vi "Swerve Drive.vi"(0 "X":dbl, 1 "Rot. Point X":dbl, 3 "Rot. Point Y":dbl, 5 "Y":dbl, 7 "Z":dbl, 11 "Error In":errorcluster, 12 "Robot Centric?":bool=TRUE, 13 "Autonomous?":bool, 14 "Yaw":dbl) -> (4 "Front Left Output":dbl, 6 "Front Right Output":dbl, 8 "Back Left Output":dbl, 10 "Back Right Output":dbl, 15 "Error Out":errorcluster)   [LabVIEW 2018]
uses:
  <vilib>/Rock Robotics/WPI/ThirdParty/Phoenix-LabVIEW/Motor Controller/Controls/CTRE_Phoenix_MotorControl_ControlMode.ctl
panel:
  in  "Robot Length":dbl=33.5
  in  "Robot Width":dbl=28.5
  # "Swerve Drive Teleoperated Control\nFRC Team 34"
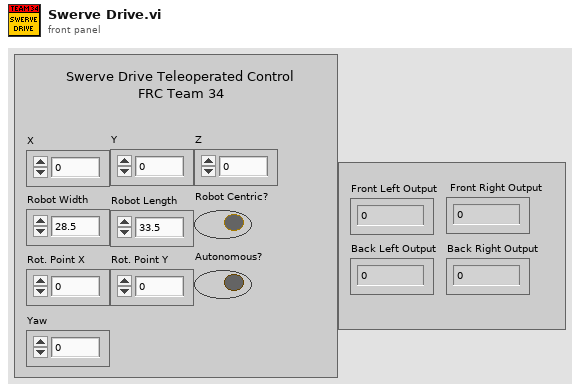
[diagram p1: front panel]
types:
  T1 = enum16{"Front Left", "Front Right", "Back Left", "Back Right"}
  T2 = typedef "CTRE_Phoenix_MotorControl_ControlMode.ctl" = u16
  T3 = typedef "WPI_MotorControlDeviceRef.ctl" = cluster{"DeviceStatus":errorcluster, "Type":T4, "PWM":cluster{"PWM Channel":T5, "DeadBand":T6}, "CAN":cluster{"Device Number":u8, "SetOutput VI Ref":variant, "GetOutput VI Ref":variant, "Enable VI Ref":variant, "Disable VI Ref":variant, "Data":variant}, "Invert":bool, "DIO PWM":cluster{"PWM \"Enable\" Channel":T5, "DIOChannel":T7, "PWM Rate":dbl}}
  T4 = typedef "WPI_MotorControlType.ctl" = enum16{"PWM", "CAN", "DIO PWM"}
  T5 = typedef "FPGA_DIOPWMChannel.ctl" = enum8{"PWM 0", "PWM 1", "PWM 2", "PWM 3", "PWM 4", "PWM 5", "PWM 6", "PWM 7", "PWM 8", "PWM 9", "PWM MXP 0", "PWM MXP 1", "PWM MXP 2", "PWM MXP 3", "PWM MXP 4", "PWM MXP 5", "PWM MXP 6", "PWM MXP 7", "PWM MXP 8", "PWM MXP 9", "Invalid"}
  T6 = typedef "WPI_PWMDeadband.ctl" = cluster{"Name":string, "maxPositivePwm":i32, "minPositivePwm":i32, "centerPwm":i32, "maxNegativePwm":i32, "minNegativePwm":i32, "angularRange":u16}
  T7 = typedef "FPGA_DIOChannel.ctl" = enum8{"DIO 0", "DIO 1", "DIO 2", "DIO 3", "DIO 4", "DIO 5", "DIO 6", "DIO 7", "DIO 8", "DIO 9", "DIO MXP 0", "DIO MXP 1", "DIO MXP 2", "DIO MXP 3", "DIO MXP 4", "DIO MXP 5", "DIO MXP 6", "DIO MXP 7", "DIO MXP 8", "DIO MXP 9", "DIO MXP 10", "DIO MXP 11", "DIO MXP 12", "DIO MXP 13", "DIO MXP 14", "DIO MXP 15", "SPI Port CS1", "SPI Port CS2", "SPI Port CS3", "SPI Port MISO", "SPI Port MOSI", "Invalid"}
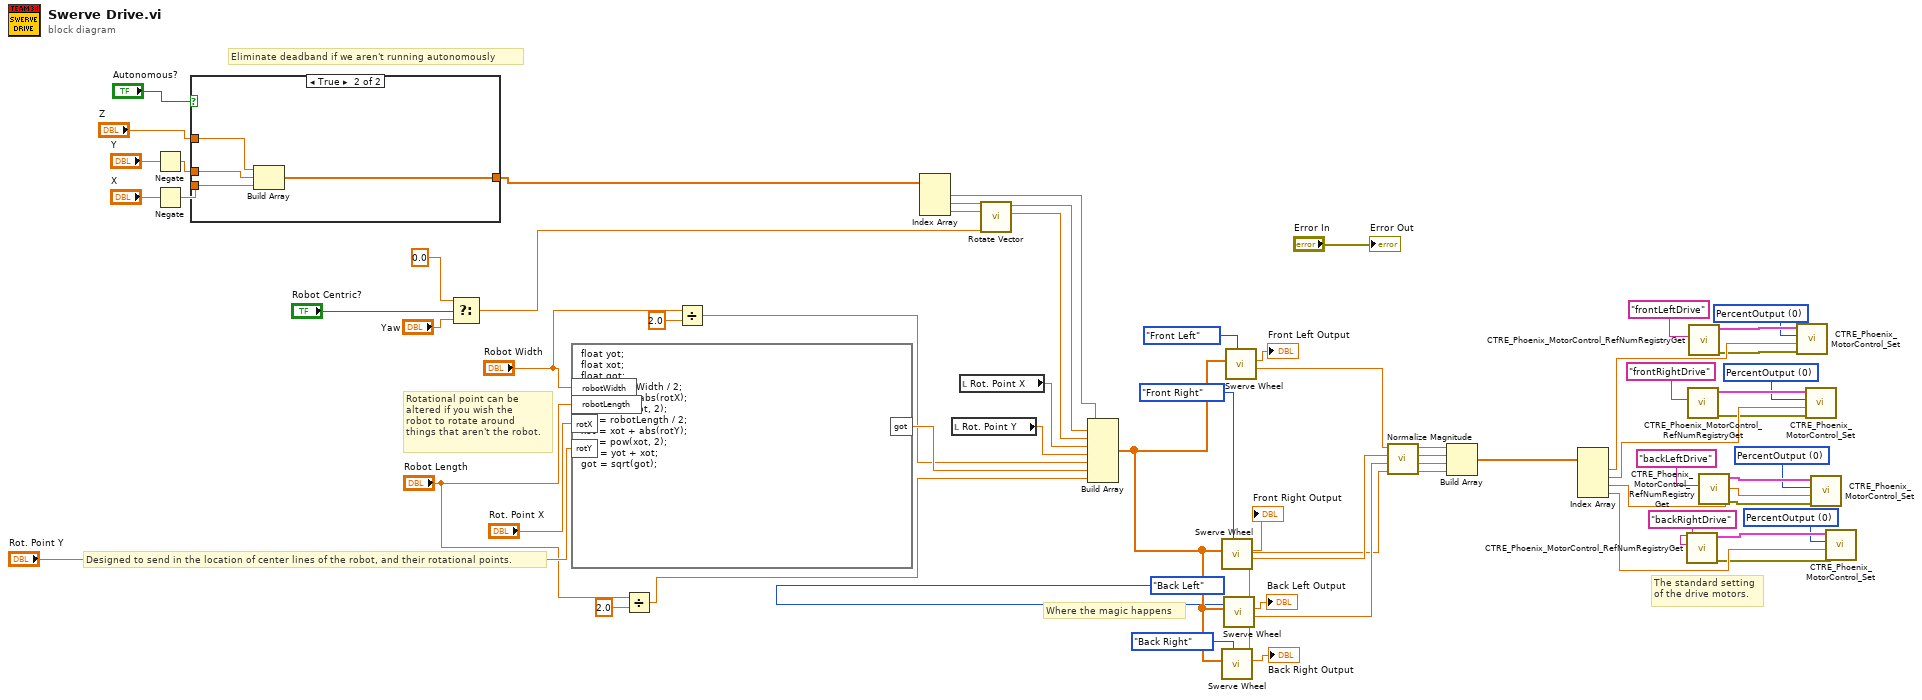
[diagram p0: block diagram]
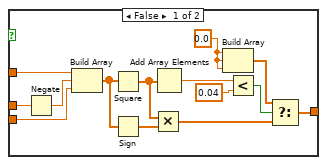
[diagram p2: hidden frame]
diagram:
  w16 = T2 0 items=["PercentOutput"=0, "Position"=1, "Velocity"=2, "Current"=3, "Follower"=5, "MotionProfile"=6, "MotionMagic"=7, "MotionMagicArc"=8, "MotionProfileArc"=10, "Disabled"=15] ("Control Mode")
  w17 = T2 0 items=["PercentOutput"=0, "Position"=1, "Velocity"=2, "Current"=3, "Follower"=5, "MotionProfile"=6, "MotionMagic"=7, "MotionMagicArc"=8, "MotionProfileArc"=10, "Disabled"=15] ("Control Mode")
  w18 = T2 0 items=["PercentOutput"=0, "Position"=1, "Velocity"=2, "Current"=3, "Follower"=5, "MotionProfile"=6, "MotionMagic"=7, "MotionMagicArc"=8, "MotionProfileArc"=10, "Disabled"=15] ("Control Mode")
  w19 = T2 0 items=["PercentOutput"=0, "Position"=1, "Velocity"=2, "Current"=3, "Follower"=5, "MotionProfile"=6, "MotionMagic"=7, "MotionMagicArc"=8, "MotionProfileArc"=10, "Disabled"=15] ("Control Mode")
  # "Rotational point can be \naltered if you wish the \nrobot to rotate around \nthings that aren't the robot."
  # "Eliminate deadband if we aren't running autonomously"
  # "Where the magic happens"
  # "The standard setting\nof the drive motors."
  # "Designed to send in the location of center lines of the robot, and their rotational points."
  n1 = Negate(x="Y") -> (-x=w37:dbl)
  n2 = Negate(x="X") -> (-x=w36:dbl)
  n3 = case shown="True" "Autonomous?" {
    tunnel: w37 -> [w70 w81]
    tunnel: [w69 w82] -> w65
    tunnel: "Z" -> [w68 w84]
    tunnel: w36 -> [w67 w83]
    frame False {
      w76 = 0.0 ("element")
      n4 = Negate(x=w70) -> (-x=w72:dbl)
      n5 = Build Array(w68, w72, w67) -> (w75:dbl[])
      n6 = Square(x=w75) -> (x^2=w73:dbl[])
      n7 = Sign(1:w75) -> (0:w74:dbl[])
      n8 = Multiply(x=w73, y=w74) -> (x*y=w71:dbl[])
      n9 = Add Array Elements(numeric array=w73) -> (sum=w80:dbl)
      n10 = Build Array(w76, w76, w76) -> (w77:dbl[])
      n11 = Less?(x=w80, y=0.04 ("x")) -> (x < y?=w78:bool)
      n12 = Select(t=w77, s=w78, f=w71) -> (s? t:f=w69:dbl[])
    }
    frame True {
      n13 = Build Array(w84, w81, w83) -> (w82:dbl[])
    }
  }
  n14 = Select(t=0.0, s="Robot Centric?", f="Yaw") -> (s? t:f=w58:dbl)
  n15 = formula code="float yot;\nfloat xot;\nfloat got;\nyot = robotWidth / 2;\nyot = yot + abs(rotX);\nyot = pow(yot, 2);\nxot = robotLength / 2;\nxot = xot + abs(rotY);\nxot = pow(xot, 2);\ngot = yot + xot;\ngot = sqrt(got);"("robotWidth"="Robot Width", "robotLength"="Robot Length", "rotX"="Rot. Point X", "rotY"="Rot. Point Y") -> ("got"=w7:dbl)
  n16 = Divide(x="Robot Length", y=2.0) -> (x/y=w4:dbl)
  n17 = Divide(x="Robot Width", y=2.0) -> (x/y=w3:dbl)
  n18 = Index Array(array=w65) -> (element #1=w57:dbl, element #2=w60:dbl, element #3=w59:dbl)  [unwired: 3 in]
  n19 = local read "Rot. Point Y"() -> (w53:dbl)
  n20 = local read "Rot. Point X"() -> (w54:dbl)
  n21 = call "Rotate Vector.vi"("Angle"=w58, "X"=w59, "Y"=w60) -> ("X'"=w55:dbl, "Y'"=w56:dbl)  [unwired: 7 in]
  n22 = Build Array(w57, w56, w55, w54, w53, w3, w7, w4) -> (w52:dbl[])
  n23 = call "Swerve Wheel.vi"("Wheel"=T1."Front Right", "Inputs"=w52) -> ("Speed"=w48:dbl, "Motor Output"=→"Front Right Output":dbl)  [unwired: 8 in]
  n24 = call "Swerve Wheel.vi"("Wheel"=T1."Back Right", "Inputs"=w52) -> ("Speed"=w46:dbl, "Motor Output"=→"Back Right Output":dbl)  [unwired: 8 in]
  n25 = call "Swerve Wheel.vi"("Wheel"=T1."Back Left", "Inputs"=w52) -> ("Speed"=w47:dbl, "Motor Output"=→"Back Left Output":dbl)  [unwired: 8 in]
  n26 = call "Swerve Wheel.vi"("Wheel"=T1."Front Left", "Inputs"=w52) -> ("Speed"=w49:dbl, "Motor Output"=→"Front Left Output":dbl)  [unwired: 8 in]
  n27 = call "Normalize Magnitude.vi"("D"=w46, "C"=w47, "B"=w48, "A"=w49) -> ("D'"=w42:dbl, "C'"=w43:dbl, "B'"=w44:dbl, "A'"=w45:dbl)  [unwired: 4 in]
  n28 = Build Array(w45, w44, w43, w42) -> (w10:dbl[])
  n29 = Index Array(array=w10) -> (element #1=w30:dbl, element #2=w24:dbl, element #3=w21:dbl, element #4=w27:dbl)  [unwired: 4 in]
  n30 = call <vilib>:"CTRE_Phoenix_MotorControl_RefNumRegistryGet.vi"("refnum name"="backRightDrive") -> ("error out"=w26:errorcluster, "PhoenixMotorControlDevRef"=w28:T3)  [unwired: 9 in]
  n31 = call <vilib>:"CTRE_Phoenix_MotorControl_RefNumRegistryGet.vi"("refnum name"="frontRightDrive") -> ("error out"=w23:errorcluster, "PhoenixMotorControlDevRef"=w25:T3)  [unwired: 9 in]
  n32 = call <vilib>:"CTRE_Phoenix_MotorControl_RefNumRegistryGet.vi"("refnum name"="frontLeftDrive") -> ("error out"=w29:errorcluster, "PhoenixMotorControlDevRef"=w31:T3)  [unwired: 9 in]
  n33 = call <vilib>:"CTRE_Phoenix_MotorControl_RefNumRegistryGet.vi"("refnum name"="backLeftDrive") -> ("error out"=w20:errorcluster, "PhoenixMotorControlDevRef"=w22:T3)  [unwired: 9 in]
  n34 = call <vilib>:"CTRE_Phoenix_MotorControl_Set.vi"("error in (no error)"=w29, "Output"=w30, "Control Mode"=w19, "PhoenixMotorControlDevRef"=w31) -> ()  [unwired: 6 in, 2 out]
  n35 = call <vilib>:"CTRE_Phoenix_MotorControl_Set.vi"("error in (no error)"=w23, "Output"=w24, "Control Mode"=w18, "PhoenixMotorControlDevRef"=w25) -> ()  [unwired: 6 in, 2 out]
  n36 = call <vilib>:"CTRE_Phoenix_MotorControl_Set.vi"("error in (no error)"=w20, "Output"=w21, "Control Mode"=w17, "PhoenixMotorControlDevRef"=w22) -> ()  [unwired: 6 in, 2 out]
  n37 = call <vilib>:"CTRE_Phoenix_MotorControl_Set.vi"("error in (no error)"=w26, "Output"=w27, "Control Mode"=w16, "PhoenixMotorControlDevRef"=w28) -> ()  [unwired: 6 in, 2 out]
  "Error Out" <- "Error In"
